vi "Pic Analysis.vi"(0 "Image in":T1, 1 "Bottom":cluster{"上边缘设置：":i32, "右边缘设置：":i32}, 3 "Top":cluster{"下边缘设置：":i32, "右边缘设置：":i32}, 11 "error in":errorcluster, 12 "Temp":T1[](array[plugin-control])) -> (4 "Image":T1(plugin-control), 6 "Centre":dbl[][](array[numeric]) format="%.2f", 8 "Found":bool, 13 "Angle":sgl, 14 "Position":sgl[](array[numeric]), 15 "错误输出":errorcluster)   [LabVIEW 2016]
uses:
  <vilib>/vision/Image Controls.llb/IMAQ Image.ctl
  <vilib>/vision/NI_Vision_Development_Module.lvlib
panel:
  in  "File Path":path=path "E:/项目/SIEMENS/图片/sd卡槽/n.bmp"
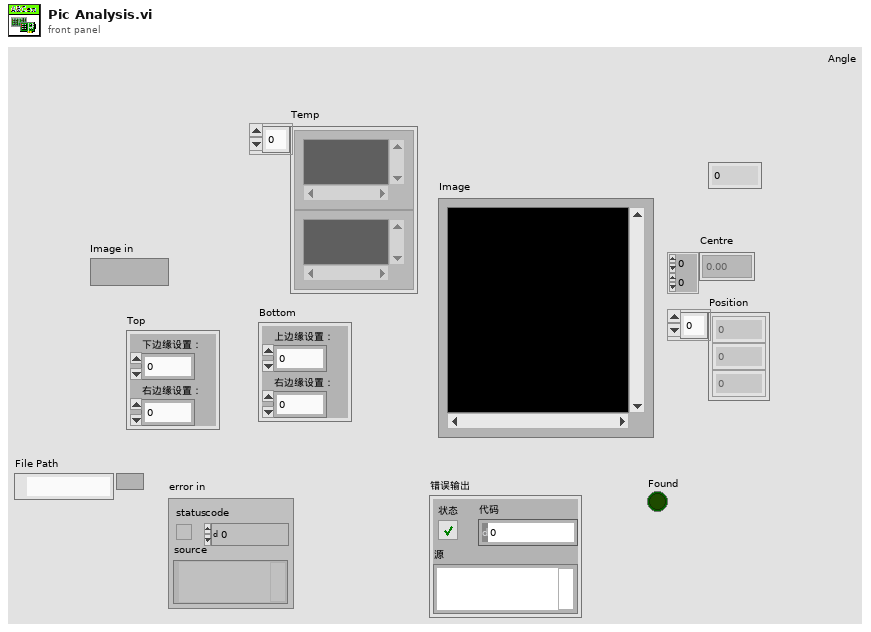
[diagram p1: front panel]
types:
  T1 = typedef "IMAQ Image.ctl" = refnum<image>
  T2 = cluster{"Global Rectangle":i32[], "Contours":cluster{"ID":enum32{"External", "Internal"}, "Type":u32, "Coordinates":i32[]}[]}
  T3 = cluster{"Algorithm":i32, "Number of Matches Requested":i32, "Minimum Match Score":sgl, "SubPixel Accuracy":bool, "Rotation Angle Ranges":cluster{"Start":sgl, "End":sgl}[], "Show Search Area":bool, "Show Result":bool}
  T4 = cluster{"Position":cluster{"x":sgl, "y":sgl}, "Angle":sgl, "Scale":sgl, "Score":sgl, "Bounding Box":cluster{"x":sgl, "y":sgl}[]}[]
  T5 = cluster{"Global Rectangle[0]":i32, "Global Rectangle[1]":i32, "Global Rectangle[2]":i32, "Global Rectangle[3]":i32}
  T6 = cluster{"Position":cluster{"x":sgl, "y":sgl}, "Angle":sgl, "Scale":sgl, "Score":sgl, "Bounding Box":cluster{"x":sgl, "y":sgl}[]}
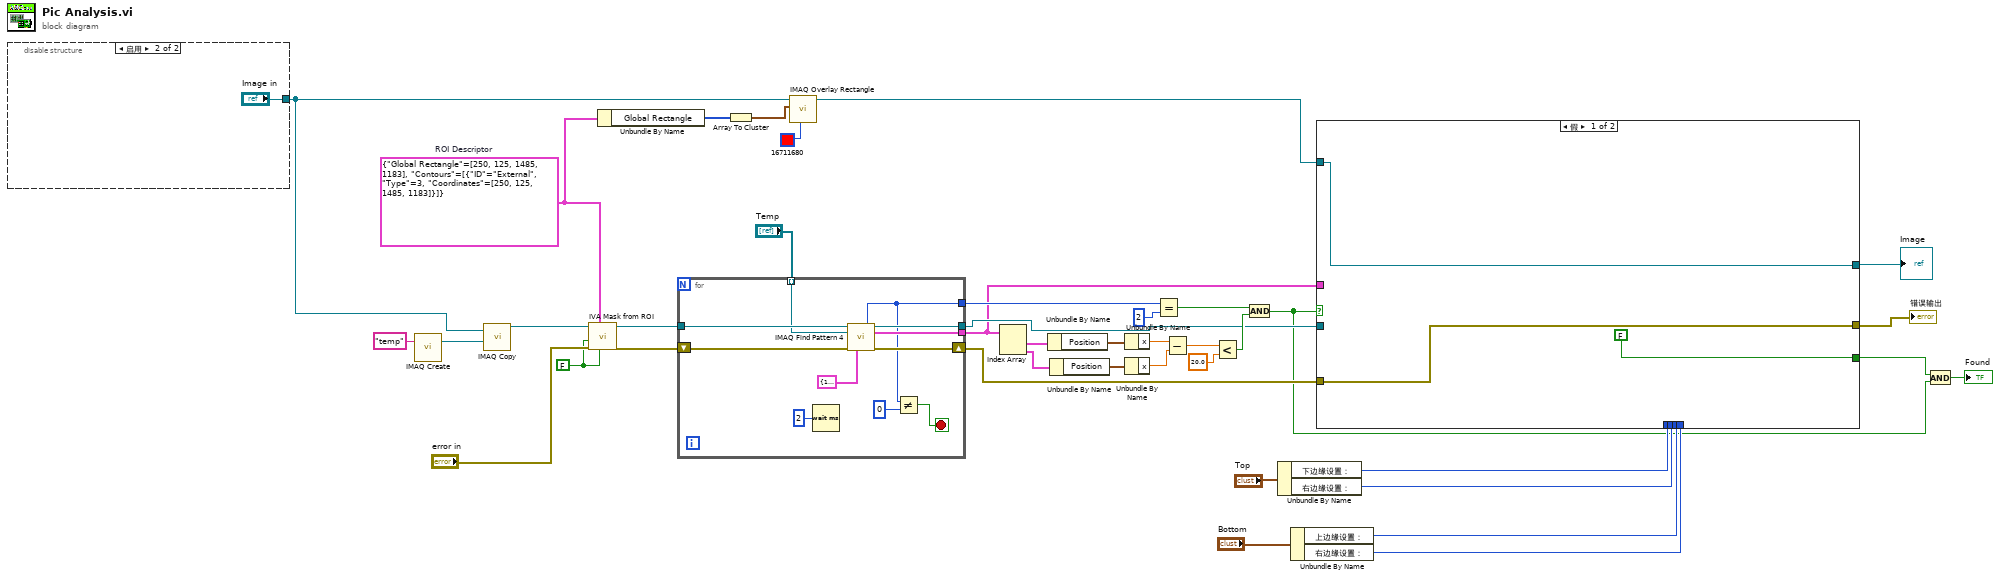
[diagram p0: block diagram]
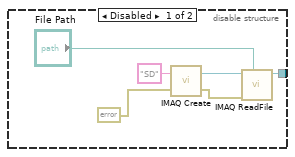
[diagram p2: hidden frame]
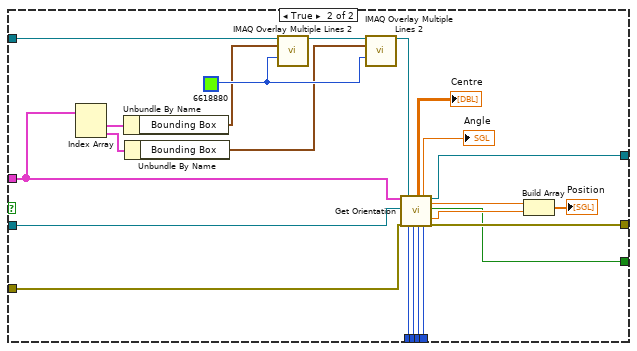
[diagram p3: hidden frame]
diagram:
  w6 = T2 {"Global Rectangle"=[250, 125, 1485, 1183], "Contours"=[{"ID"=enum."External", "Type"=3, "Coordinates"=[250, 125, 1485, 1183]}]}  # ROI Descriptor
  w11 = FALSE
  n1 = disable-structure shown="启用" {
    disable-tunnel: [w42 "Image in"] -> w7
    frame Disabled {
      n2 = call "IMAQ Create"("Image Name"="SD", "error in (no error)"=errorcluster {"status"=FALSE, "code"=0, "source"=""}) -> ("New Image"=w44:T1, "error out"=w43:errorcluster)  [unwired: 3 in]
      n3 = call "IMAQ ReadFile"("File Path"="File Path", "error in (no error)"=w43, "Image"=w44) -> ("Image Out"=w42:T1)  [unwired: 4 in, 4 out]
    }
    frame Enabled {
    }
  }
  n4 = call "IMAQ Create"("Image Name"="temp") -> ("New Image"=w10:T1)  [unwired: 4 in, 1 out]
  n5 = call "IMAQ Copy"("Image Dst"=w10, "Image Src"=w7) -> ("Image Dst Out"=w8:T1)  [unwired: 4 in, 1 out]
  n6 = call <vilib>:"IVA Mask from ROI.vi"("Shrink"=w11, "ROI Descriptor"=w6, "error in (no error)"="error in", "Out / In"=w11, "Image Src"=w8) -> ("error out"=w13:errorcluster, "Image Out"=w12:T1)  [unwired: 5 out]
  n7 = Unbundle By Name(w6) -> ("Global Rectangle"=w5:i32[])
  n8 = for {
    tunnel: [w55] -> w2
    tunnel: [w50] -> w27
    shift-right: [w54] -> w28
    shift-left: w13 -> [w53]
    tunnel: "Temp" -> [w52] mode=indexing
    tunnel: w12 -> [w58]
    tunnel: [w56] -> w29
    stop <- w51 stop-if-true
    n9 = Wait (ms)(milliseconds to wait=u32 2 ("等待时间（毫秒）")) -> ()  [unwired: 1 out]
    n10 = call "IMAQ Find Pattern 4"("Image"=w58, "Template"=w52, "error in"=w53, "Settings"=T3 {"Algorithm"=1, "Number of Matches Requested"=2, "Minimum Match Score"=700.0, "SubPixel Accuracy"=FALSE, "Rotation Angle Ranges"=[{"Start"=-2.0, "End"=2.0}], "Show Search Area"=FALSE, "Show Result"=TRUE}) -> ("Number of Matches"=w50:i32, "Image Out"=w56:T1, "Matches (pixel)"=w55:T4, "error out"=w54:errorcluster)  [unwired: 5 in, 3 out]
    n11 = Not Equal?(x=w50, y=0) -> (x != y?=w51:bool)
  }
  n12 = Array To Cluster(array=w5) -> (cluster=w4:T5)
  n13 = call "IMAQ Overlay Rectangle"("Color"=u32 16711680, "Rectangle"=w4, "Image"=w7) -> ("Image Out"=w1:T1)  [unwired: 7 in, 1 out]
  n14 = Index Array(array=w2) -> (element #1=w40:T6, element #2=w39:T6)  [unwired: 2 in]
  n15 = Unbundle By Name(w40) -> ("Position"=w38:cluster{"x":sgl, "y":sgl})
  n16 = Unbundle By Name(w39) -> ("Position"=w37:cluster{"x":sgl, "y":sgl})
  n17 = Unbundle By Name(w38) -> ("x"=w36:sgl)
  n18 = Unbundle By Name(w37) -> ("x"=w35:sgl)
  n19 = Equal?(x=w27, y=2) -> (x = y?=w31:bool)
  n20 = Subtract(x=w36, y=w35) -> (x-y=w34:sgl)
  n21 = Less?(x=w34, y=sgl 20.0) -> (x < y?=w30:bool)
  n22 = And(x=w31, y=w30) -> (x .and. y?=w15:bool)
  n23 = Unbundle By Name("Top") -> ("下边缘设置："=w25:i32, "右边缘设置："=w24:i32)
  n24 = Unbundle By Name("Bottom") -> ("上边缘设置："=w22:i32, "右边缘设置："=w21:i32)
  n25 = case shown="假" w15 {
    tunnel: w29 -> [_ w72]
    tunnel: w2 -> [_ w64]
    tunnel: w28 -> [w61 w84]
    tunnel: w25 -> [_ w82]
    tunnel: w24 -> [_ w81]
    tunnel: w22 -> [_ w80]
    tunnel: w21 -> [_ w79]
    tunnel: [w61 w78] -> w20
    tunnel: [w59 w74] -> w19
    tunnel: [FALSE ("no error") w73] -> w16
    tunnel: w1 -> [w59 w68]
    frame False {
    }
    frame True {
      w70 = u32 6618880
      n26 = Index Array(array=w64) -> (element #1=w65:T6, element #2=w66:T6)  [unwired: 2 in]
      n27 = Unbundle By Name(w65) -> ("Bounding Box"=w63:cluster{"x":sgl, "y":sgl}[])
      n28 = Unbundle By Name(w66) -> ("Bounding Box"=w62:cluster{"x":sgl, "y":sgl}[])
      n29 = call "IMAQ Overlay Multiple Lines 2"("Image"=w68, "Line End Points"=w63, "Color"=w70) -> ("Image Out"=w69:T1)  [unwired: 11 in, 1 out]
      n30 = call "IMAQ Overlay Multiple Lines 2"("Image"=w69, "Line End Points"=w62, "Color"=w70) -> ("Image Out"=w67:T1)  [unwired: 11 in, 1 out]
      n31 = call "Get Orientation.vi"("Matches (pixel)"=w64, "Image Src"=w72, "error in (no error)"=w84, "Image Dst"=w67, "y"=w82, "X"=w81, "yB"=w80, "XB"=w79) -> ("Centre"=→"Centre":dbl[][], "Angle"=→"Angle":sgl, "Image 3"=w74:T1, "X"=w71:sgl, "no error"=w73:bool, "y"=w76:sgl, "错误输出"=w78:errorcluster)  [unwired: 5 in]
      n32 = Build Array(w71, w76) -> (→"Position":sgl[])
    }
  }
  "错误输出" <- w20
  "Image" <- w19
  n33 = Compound Arithmetic op=AND ("复合运算")(w16, w15) -> (→"Found":bool)
